vi "Dashboard Main.vi"() -> ()   [LabVIEW 2018]
uses:
  <vilib>/Utility/miscctls.llb/LVRowAndColumnTypeDef.ctl
  <vilib>/event_ctls.llb/eventvkey.ctl
  <vilib>/Rock Robotics/Network Tables/NT Read Boolean.vi
  <vilib>/Rock Robotics/Network Tables/NT Write Boolean.vi
  <vilib>/Rock Robotics/Network Tables/NT Read Numeric Array.vi
  <vilib>/Rock Robotics/WPI/Dashboard/WPI_DashboardLogging Global.vi
panel:
  in  "Camera Settings Right":T1={"Frame Rate"=30, "Compression"=30, "Size"=1, "DB Camera Config"=FALSE} {"Frame Rate" scale=1.0..30.0; "Compression" scale=100.0..-1.0; "Size" items=["640x480", "320x240", "160x120"]}
  in  "Camera Name Right":string(combo)="No Camera Selection"
  out "Camera Perf":string
  in  "Camera Settings":T1={"Frame Rate"=30, "Compression"=30, "Size"=1, "DB Camera Config"=FALSE} {"Frame Rate" scale=1.0..30.0; "Compression" scale=100.0..-1.0; "Size" items=["640x480", "320x240", "160x120"]}
  in  "TCP":refnum<k5>
  in  "Rec Mode":enum32{"Stop", "Record", "Playback"}(radio)
  out "Image Message":string="Timeout in Camera Communications"
  in  "Dashboard Tab":T2(tab)
  out "Lift Height":dbl
  in  "Auto Side":bool
  out "Limelight Target State":bool
  out "Hatch Open":bool
  out "Hatch Extend":bool
  out "Cargo Piston":bool
  in  "Zero Yaw":bool
  out "Yaw":dbl
  out "Cont Yaw":dbl
  out "LowerLimit":bool
  out "UpperLimit":bool
  out "HAB Retracting limit":bool
  out "HAB Extending limit":bool
  in  "Select Auto":string(combo)="Select Autonomous ..."
  out "NT Connection":bool
  out "Mode":T3(ring)=enum."Auto Disabled"
  out "Right Camera Perf":cluster{"Bandwidth (Mbps)":dbl, "FPS":dbl}
  out "Lift Auto Position":u16(ring) items=["Cargo 1", "Hatch 1", "Cargo 2", "Hatch 2", "Cargo 3", "Hatch 3"]
  out "CargoLimit":bool
  out "Wheel Rates":T4
  out "Wheel Angles":T4
  out "Y-Velocity":dbl
  out "X-Velocity":dbl
  out "Wheel Positions":T4
  in  "Starting Location":u16(ring)=2 items=["Left", "Center", "Right"]
  out "Positions":cluster{"X":dbl, "Y":dbl}
  out "Graph 2":cluster{cluster{"X":dbl, "Y":dbl}[]}[](graph)=[{[{"X"=44.0, "Y"=76.0}, {"X"=44.0, "Y"=76.0}]}, {[{"X"=30.03458329904793, "Y"=57.973155118857626}, {"X"=30.03458329904793, "Y"=57.973155118857626}]}, {[{"X"=29.965468303127132, "Y"=93.97308877320398}, {"X"=29.965468303127132, "Y"=93.97308877320398}]}, {[{"X"=57.96541670095207, "Y"=94.02684488114238}, {"X"=57.96541670095207, "Y"=94.02684488114238}]}, {[{"X"=58.03453169687287, "Y"=58.026911226796024}, {"X"=58.03453169687287, "Y"=58.026911226796024}]}, {[{"X"=43.942404170066, "Y"=105.9999447119553}, {"X"=43.942404170066, "Y"=105.9999447119553}]}]
  out "Tree":string(tree)
  in  "Test Slider":dbl(slide) scale=0.0..100.0 scale format="%#_3g"
  in  "On/Off":bool caption="Solenoid"
  in  "Test Name":u16(ring) items=["Select the test to run..."]
  in  "Test Tree":string(tree)
  in  "Motor":cluster{"Value":dbl, "Enable":bool} {"Value" scale=-1.0..1.0 scale format="%#_3g"}
  out "Progress":T5 {"Test Progress" scale=0.0..100.0}
  in  "Rev/Fwd":cluster{"Forward":bool, "Reverse":bool}
  in  "Test Ring":u16(ring) items=["Monochrome", "Color"]
  in  "CheckList":i32(listbox)
  out "Cmd Status":string
  in  "Execute Command":bool
  in  "Command Params":string[][](table)
  in  "Command Selection":i32(listbox)
  out "Camera Image":T6(plugin-control)
  in  "Camera Name":string(combo)="No Camera Selection"
  # "HW"
  # "HW"
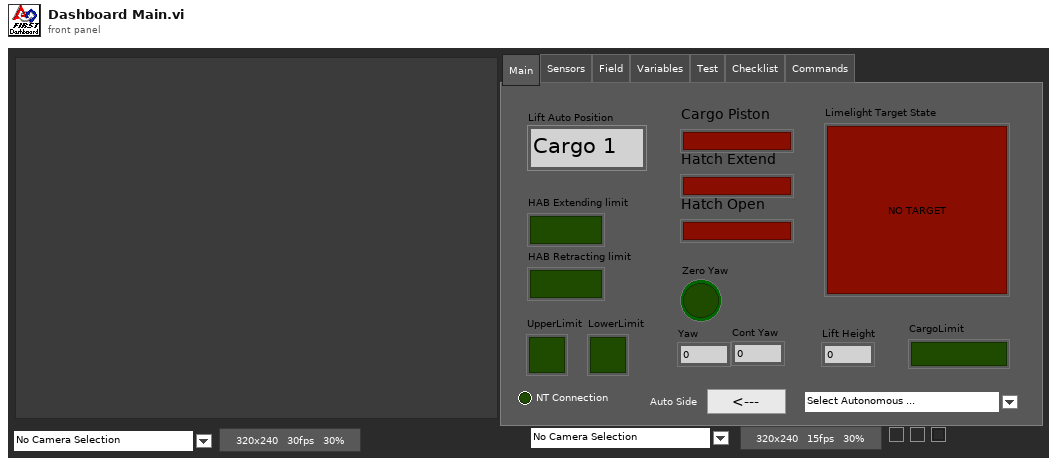
[diagram p1: front panel]
types:
  T1 = cluster{"Frame Rate":i32, "Compression":i32, "Size":u16, "DB Camera Config":bool}
  T2 = enum32{"Main", "Sensors", "Field", "Variables", "Test", "Checklist", "Commands"}
  T3 = enum8{"Tele-Op Disabled", "Tele-Op Enabled", "Auto Disabled", "Auto Enabled", "Test Disabled", "Test Enabled", "Disconnected", "No Code", "E-Stop"}
  T4 = cluster{"FrontLeft":dbl, "FrontRight":dbl, "BackLeft":dbl, "BackRight":dbl}
  T5 = cluster{"Test Progress":u8, "Test Progress Text":string}
  T6 = typedef "IMAQ Image.ctl" = refnum<image>
  T7 = cluster{"Save Path":path, "Interval (s)":dbl, "Keep":i32}
  T8 = enum32{"Drive", "Camera", "Basic", "Custom", "Test", "Commands", "Checklist", "Variables"}
  T9 = typedef "Image Type" = u32
  T10 = cluster{"IDs":cluster{"RPC field ID":u16, "Unique ID":u16}, "String":string}
  T11 = cluster{"Error Strings":string, "Disable Counts":cluster{u16, u16}, "Rail Faults":cluster{u16, u16, u16}, "Robot IP":string, "DB Mode":u8, "Event Info":cluster{"Name":string, "Type":u8, "Number":u16, "Replay":u8}}
  T12 = cluster{"Storage":cluster{"Disk Free":u64, "RAM Block":u32, "RAM free":u32}, "CPU Utilization":cluster{"CPU % ISR":sgl, "CPU % Time Crit":sgl, "CPU % Timed Str":sgl, "CPU % High":sgl, "CPU % Above":sgl, "CPU % Normal":sgl, "CPU % Low":sgl}, "CAN":cluster{"% Bus Utilization":sgl, "Bus Off Cnt":u32, "TX_FIFO Full Cnt":u32, "Receive Error Cnt":u8, "Transmit Error Cnt":u8}, "HID":cluster{"HID Outputs":u32, "Rumble Low":u16, "Rumble High":u16}[]}
  T13 = cluster{"Status bits":cluster{"Test Mode":bool, "Autonomous":bool, "Enabled":bool, "Code Start":bool, "Brownout":bool, "Reserved 2":bool, "Reserved 3":bool, "E-Stop":bool}, "Code Trace":cluster{"Disabled":bool, "TeleOp":bool, "Auto":bool, "Test":bool}, "Controller Type":enum16{"unknown", "cRIO", "roboRio"}, "Code?":enum16{"unknown", "noCode", "code"}, "Battery V":dbl}
  T14 = cluster{"Control Bits":cluster{"TestMode":bool, "Autonomous":bool, "Enabled":bool, "FMS Present":bool, bool, bool, bool, "E-Stop":bool}, "Team Station ":u8, "Countdown":sgl, "Joystick Values":cluster{"Axes":dbl[], "Buttons":bool[], "POVs":i16[]}[]}
  T15 = cluster{"Numeric":dbl, "Numeric":dbl, "Numeric":dbl, "Numeric":dbl}
  T16 = cluster{"Global Rectangle":i32[], "Contours":cluster{"Contour Type":u32, "ROI Type":u32, "Points":i32[]}[]}
  T17 = cluster{"Camera Name":string, string, "Saved DB Images Info":cluster{"Save Path":path, "Interval (s)":dbl, "Keep":i32}}
  T18 = cluster{"Camera Name Right":string, string, "Saved DB Images Info":cluster{"Save Path":path, "Interval (s)":dbl, "Keep":i32}}
  T19 = cluster{"Operation":enum16{"Update", "Clear"}, "Color Box":u32}[]
  T20 = typedef "eventvkey.ctl" = enum16{"ASCII", "Enter", "Return", "Shift", "Ctrl", "Alt", "Cmd", "Opt", "Caps", "NumLock", "Clear", "Break", "Up", "Down", "Left", "Right", "Insert", "Delete", "Home", "End", "PageUp", "PageDown", "Escape", "Help", "Pause", "ScrollLock", "F1", "F2", "F3", "F4", "F5", "F6", "F7", "F8", "F9", "F10", "F11", "F12", "F13", "F14", "F15", "F16", "F17", "F18", "F19", "F20", "F21", "F22", "F23", "F24", "Play", "VolumeUp", "VolumeDown", "Mute", "Two Byte Char"}
  T21 = cluster{"Operation":enum16{"Update", "Clear"}, "Color Box":u32}
  T22 = typedef "LVRowAndColumnTypeDef.ctl" = cluster{"Row":i32, "Column":i32}
  T23 = cluster{"Shift":bool, "Ctrl":bool, "Alt":bool, "Cmd":bool, "Opt":bool}
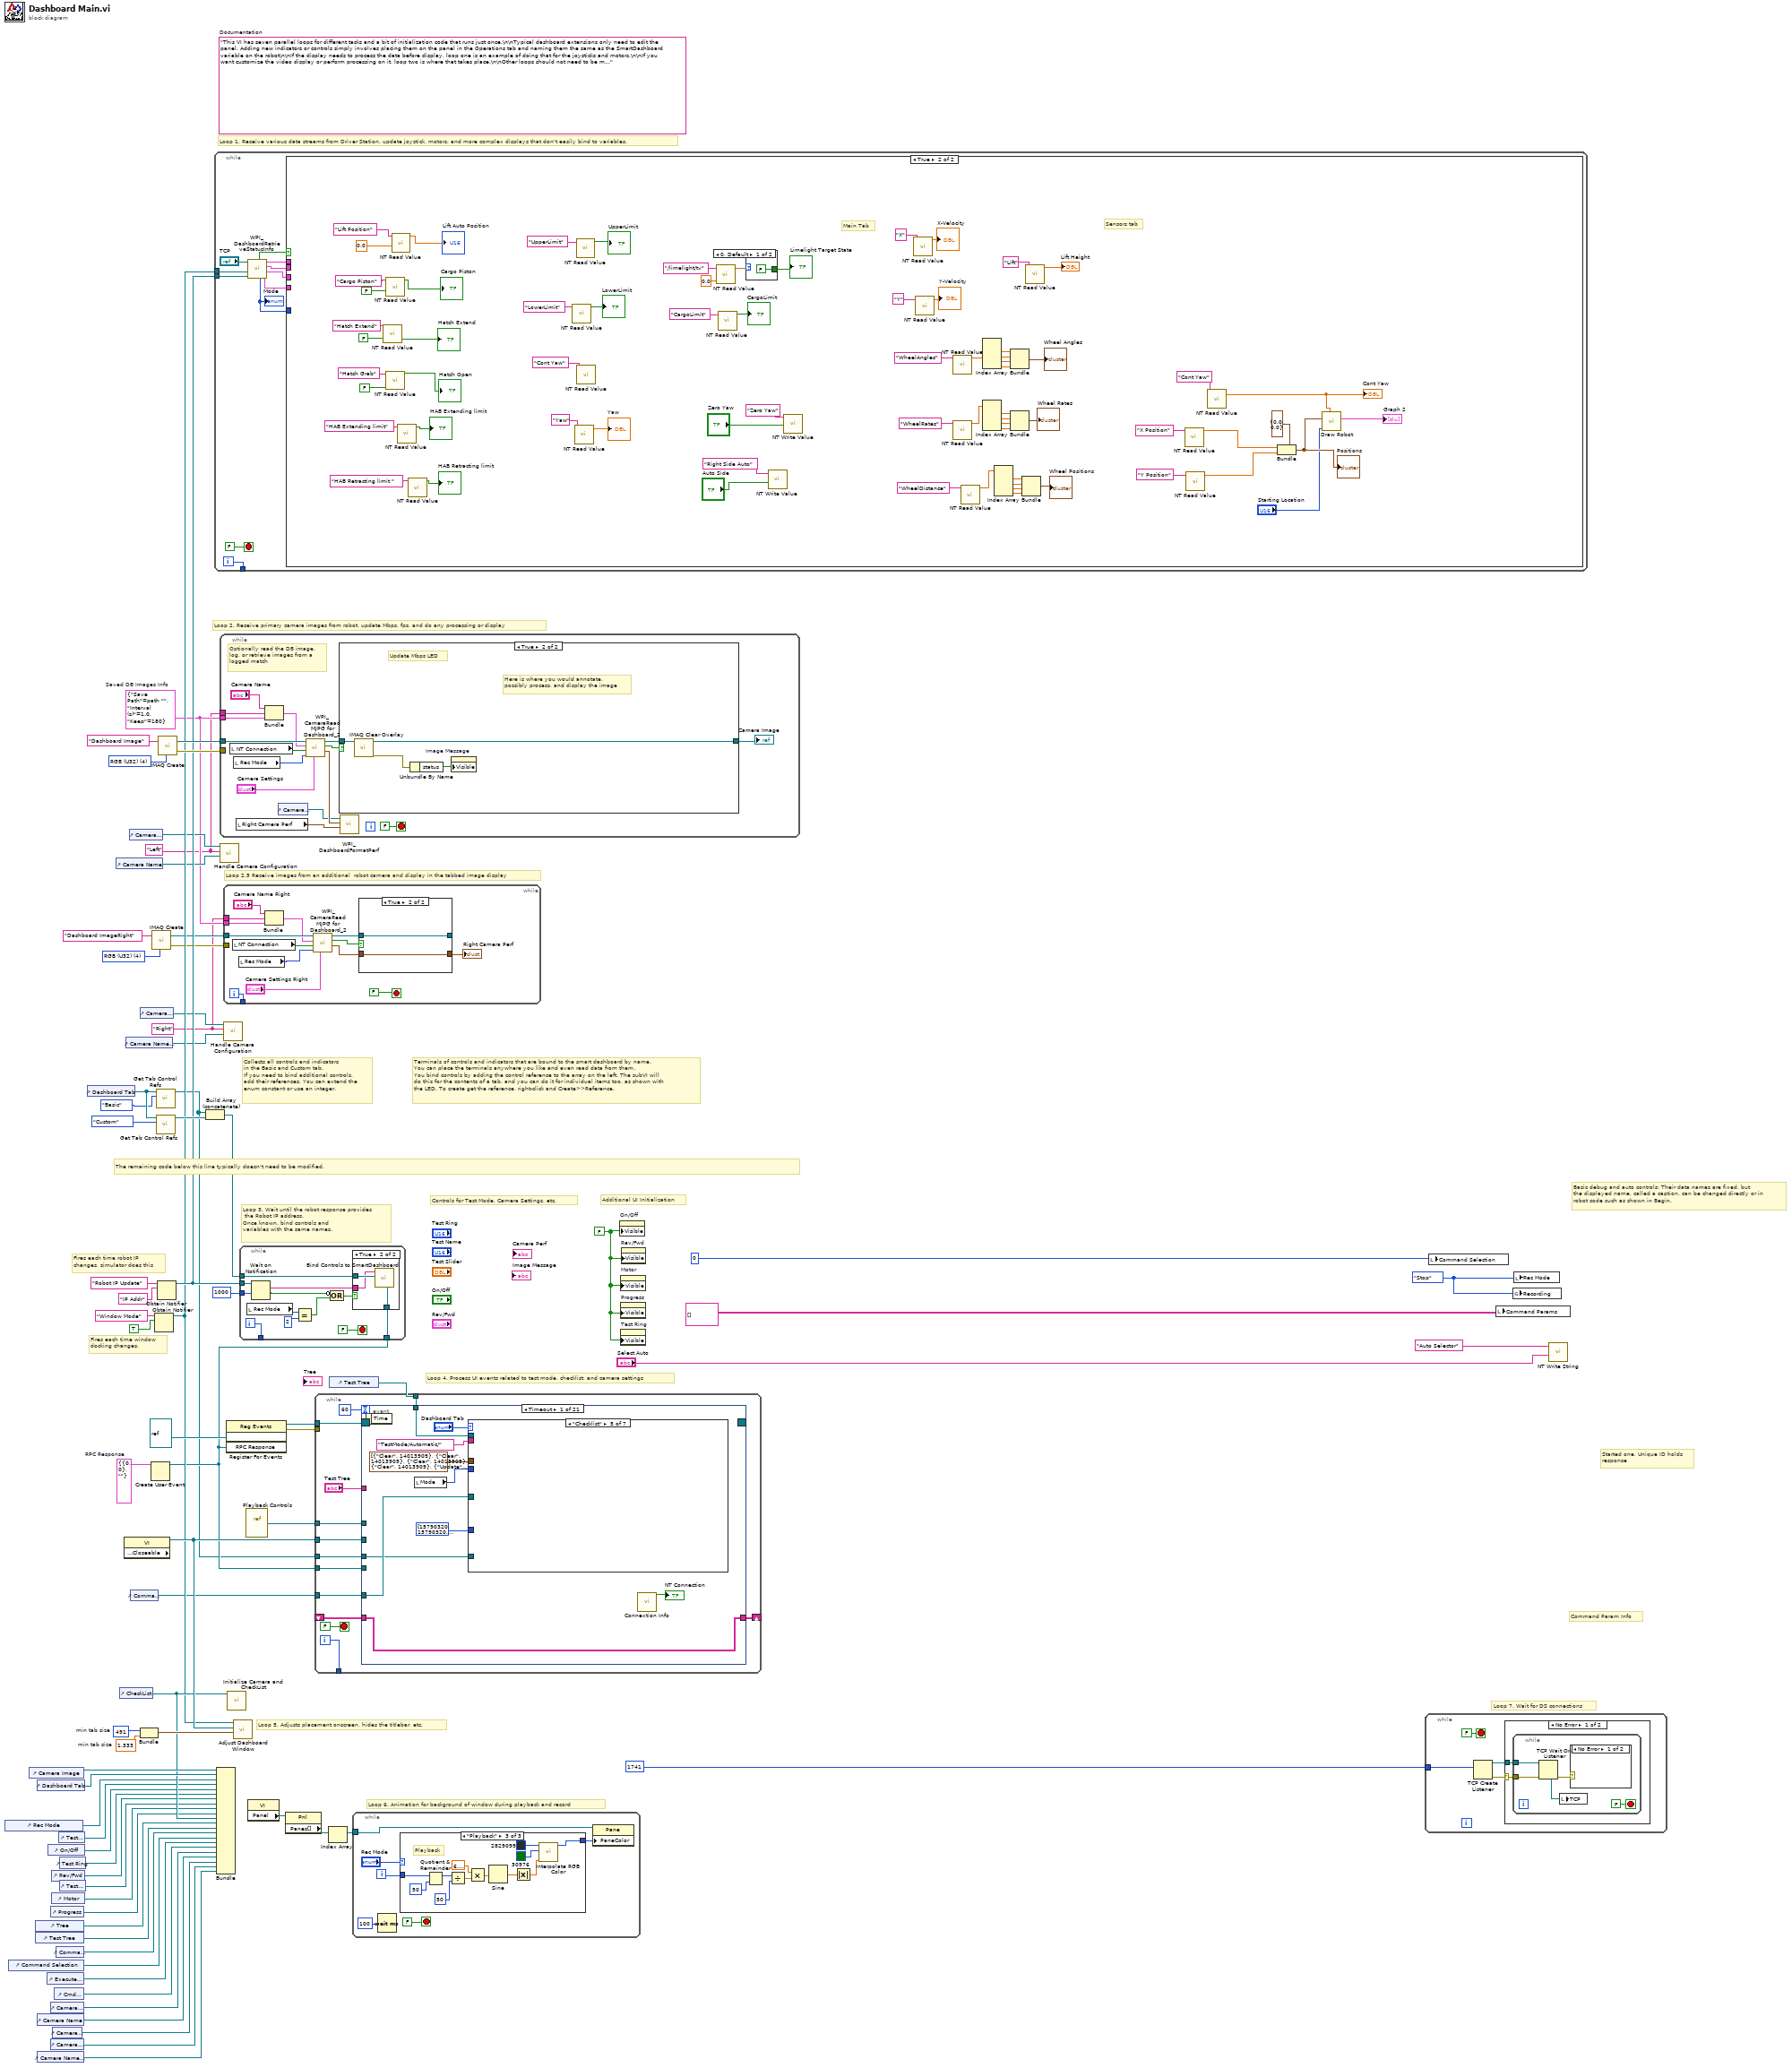
[diagram p0: block diagram]
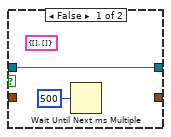
[diagram p2: hidden frame]
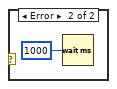
[diagram p3: hidden frame]
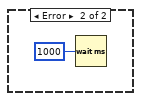
[diagram p4: hidden frame]
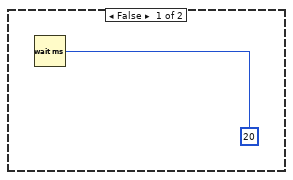
[diagram p5: hidden frame]
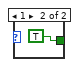
[diagram p6: hidden frame]
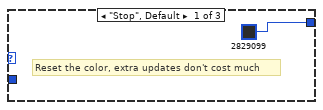
[diagram p7: hidden frame]
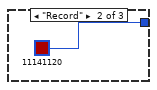
[diagram p8: hidden frame]
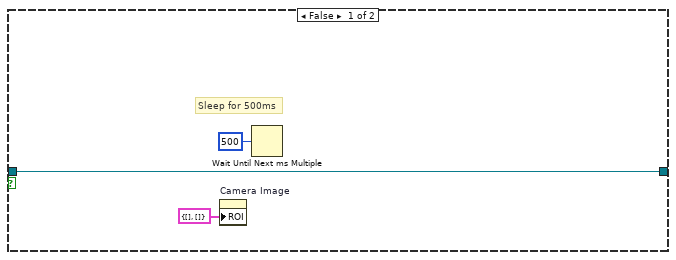
[diagram p10: hidden frame]
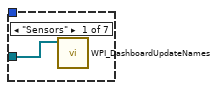
[diagram p11: hidden frame]
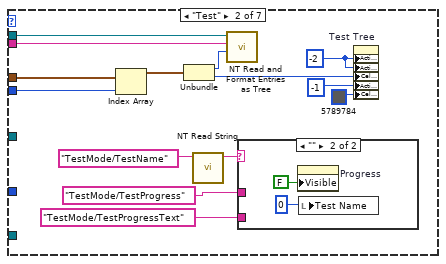
[diagram p12: hidden frame]
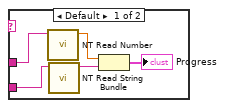
[diagram p13: hidden frame]
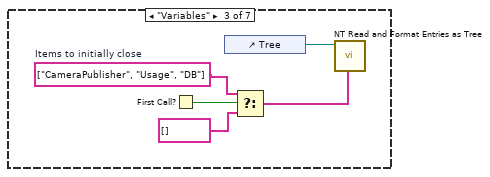
[diagram p14: hidden frame]
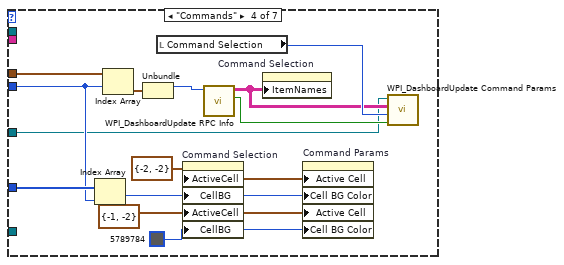
[diagram p15: hidden frame]
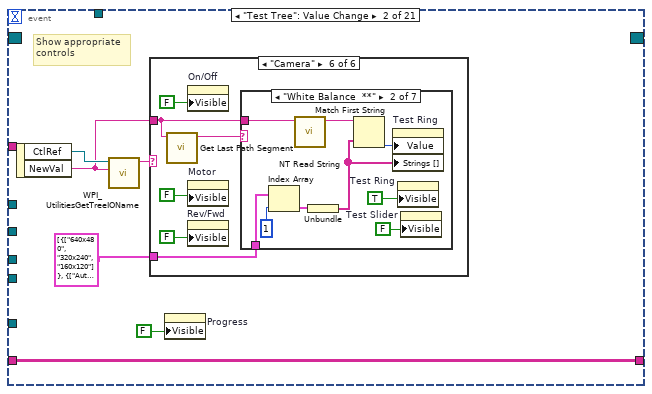
[diagram p18: hidden frame]
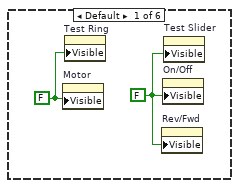
[diagram p19: hidden frame]
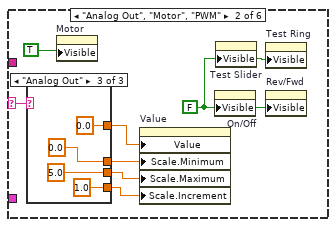
[diagram p20: hidden frame]
diagram:
  w3 = T7 {"Save Path"=path "", "Interval (s)"=1.0, "Keep"=180}  # Saved DB Images Info
  w2 = "Right"
  w1 = "Left"
  w12 = T9 4 items=["Grayscale (U8)", "Grayscale (I16)", "Grayscale (SGL)", "Complex (CSG)", "RGB (U32)", "HSL (U32)", "RGB (U64)"] ("Image Type")
  w28 = T10 {"IDs"={"RPC field ID"=0, "Unique ID"=0}, "String"=""}  # RPC Response
  w48 = 491  # min tab size
  w47 = 1.333  # min tab size
  w55 = enum32{"Stop", "Record", "Playback"}."Stop" ("Rec Mode")
  w34 = FALSE ("Visible")
  (unwired) "This VI has seven parallel loops for different tasks and a bit of initialization code that runs just once.\n\nTypical dashboard extensions only need to edit the panel. Adding new indicators or controls simply involves placing them on the panel in the Operations tab and naming them the same as the SmartDashboard variable on the robot\n\nIf the display needs to process the data before display, loop one is an example of doing that for the joysticks and motors.\n\nIf you want customize the video display or perform processing on it, loop two is where that takes place.\n\nOther loops should not need to be modified. They are pretty standard, and document the task they perform."  # Documentation
  w72 = T9 4 items=["Grayscale (U8)", "Grayscale (I16)", "Grayscale (SGL)", "Complex (CSG)", "RGB (U32)", "HSL (U32)", "RGB (U64)"] ("Image Type")
  # "Loop 2.5 Receive images from an additional  robot camera and display in the tabbed image display"
  # "Command Param Info"
  # "Started one, Unique ID holds\nresponse"
  # "Loop 7. Wait for DS connections"
  # "Basic debug and auto controls: Their data names are fixed, but\nthe displayed name, called a caption, can be changed directly or in\nrobot code such as shown in Begin."
  # "Controls for Test Mode, Camera Settings, etc."
  # "Additional UI Initialization"
  # "Loop 6. Animation for background of window during playback and record"
  # "Fires each time robot IP\nchanges, simulator does this"
  # "Fires each time window\ndocking changes."
  # "Collects all controls and indicators\nin the Basic and Custom tab.\nIf you need to bind additional controls,\nadd their references. You can extend the\nenum constant or use an integer."
  # "The remaining code below this line typically doesn't need to be modified."
  # "Loop 4. Process UI events related to test mode, checklist, and camera settings"
  # "Terminals of controls and indicators that are bound to the smart dashboard by name.\nYou can place the terminals anywhere you like and even read data from them.\nYou bind controls by adding the control reference to the array on the left. The subVI will\ndo this for the contents of a tab, and you can do it for individual items too, as shown with\nthe LED. To create get the reference, right-click and Create>>Reference."
  # "Loop 3. Wait until the robot response provides\n the Robot IP address.\nOnce known, bind controls and\nvariables with the same names."
  # "Loop 5. Adjusts placement onscreen, hides the titlebar, etc."
  # "Loop 1. Receive various data streams from Driver Station, update joystick, motors, and more complex displays that don't easily bind to variables."
  # "Loop 2. Receive primary camera images from robot, update Mbps, fps, and do any processing or display"
  n1 = control-ref of="Rec Mode"() -> (w40:refnum<vi>)
  n2 = control-ref of="Command Selection"() -> (w27:refnum<vi>)
  n3 = control-ref of="Camera Image"() -> (w50:refnum<vi>)
  n4 = control-ref of="Tree"() -> (w44:refnum<vi>)
  n5 = control-ref of="Test Tree"() -> (w43:refnum<vi>)
  n6 = control-ref of="Dashboard Tab"() -> (w49:refnum<vi>)
  n7 = control-ref of="Camera Name"() -> (w18:refnum<vi>)
  n8 = control-ref of="Camera Name Right"() -> (w6:refnum<vi>)
  n9 = control-ref of="Execute Command"() -> (w29:refnum<vi>)
  n10 = control-ref of="On/Off"() -> (w38:refnum<vi>)
  n11 = control-ref of="Progress"() -> (w35:refnum<vi>)
  n12 = control-ref of="Camera Settings"() -> (w19:refnum<vi>)
  n13 = control-ref of="Camera Settings Right"() -> (w7:refnum<vi>)
  n14 = control-ref of="Rev/Fwd"() -> (w36:refnum<vi>)
  n15 = control-ref of="Motor"() -> (w41:refnum<vi>)
  n16 = control-ref of="Camera Perf"() -> (w17:refnum<vi>)
  n17 = control-ref of="Cmd Status"() -> (w23:refnum<vi>)
  n18 = control-ref of="Command Params"() -> (w30:refnum<vi>)
  n19 = control-ref of="Test Slider"() -> (w39:refnum<vi>)
  n20 = control-ref of="Test Ring"() -> (w37:refnum<vi>)
  n21 = control-ref of="Test Name"() -> (w42:refnum<vi>)
  n22 = control-ref of="Dashboard Tab"() -> (w53:refnum<vi>)
  n23 = control-ref of="Camera Name"() -> (w20:refnum<vi>)
  n24 = control-ref of="CheckList"() -> (w45:refnum<vi>)
  n25 = property class="VI" props=["Front Panel.Closeable"]() -> (reference out=w54:refnum<vi>)  [unwired: 2 in, 2 out]
  n26 = control-ref of="Camera Name Right"() -> (w8:refnum<vi>)
  n27 = control-ref of="Camera Settings"() -> (w21:refnum<vi>)
  n28 = control-ref of="Command Params"() -> (w22:refnum<vi>)
  n29 = control-ref of="Camera Settings Right"() -> (w9:refnum<vi>)
  n30 = Bundle("min tab size"=w48, "min tab size"=w47) -> (w46:cluster{"min tab size":i32, "min tab size":dbl})  [unwired: 1 in]
  n31 = Create User Event(user event datatype=w28) -> (user event=w24:refnum<user-event>)  [unwired: 1 in, 1 out]
  n32 = call "IMAQ Create"("Image Name"="Dashboard ImageRight", "Image Type"=w12) -> ("New Image"=w11:T6, "error out"=w10:errorcluster)  [unwired: 2 in, 1 out]
  n33 = Obtain Notifier(name (unnamed)="Window Mode", notification data type=TRUE) -> (notifier out=w32:refnum<notifier>)  [unwired: 2 in, 2 out]
  n34 = call <vilib>:"Get Tab Control Refs.vi"("Page Index"=T8."Basic" ("Dashboard Tab"), "TabControl in"=w53) -> ("ControlsOnPage"=w16:refnum<vi>[])  [unwired: 9 in]
  n35 = call <vilib>:"Get Tab Control Refs.vi"("Page Index"=T8."Custom" ("Dashboard Tab"), "TabControl in"=w53) -> ("ControlsOnPage"=w52:refnum<vi>[])  [unwired: 9 in]
  n36 = Obtain Notifier(name (unnamed)="Robot IP Update", notification data type="IP Addr" ("name (unnamed)")) -> (notifier out=w33:refnum<notifier>)  [unwired: 2 in, 2 out]
  n37 = call "IMAQ Create"("Image Name"="Dashboard Image", "Image Type"=w72) -> ("New Image"=w70:T6, "error out"=w69:errorcluster)  [unwired: 2 in, 1 out]
  n38 = Build Array (concatenate)(w16, w52) -> (w51:refnum<vi>[])
  n39 = while {
    tunnel: [w82] -> _
    tunnel: w33 -> [w80]
    tunnel: w32 -> [w77]
    i -> [w82]
    stop <- FALSE stop-if-true
    n40 = call <vilib>:"WPI_DashboardRetrieveStatusInfo.vi"("Binding Refnum"=w80, "Window Mode Notifier"=w77, "TCP Cnx"="TCP") -> ("Power and Errors"=w74:T11, "Robot Metrics"=w73:T12, "Status Info"=w75:T13, "Control Info"=w76:T14, "Robot Mode"=w79:T3, "Process?"=w81:bool)  [unwired: 3 in]
    "Mode" <- w79
    n41 = case shown="True" w81 {
      tunnel: w79 -> [_ _]
      tunnel: w76 -> [_ _]
      tunnel: w75 -> [_ _]
      tunnel: w74 -> [_ _]
      tunnel: w73 -> [_ _]
      frame False {
        n42 = Wait (ms)(milliseconds to wait=u32 20) -> ()  [unwired: 1 out]
      }
      frame True {
        # "Sensors tab"
        # "Main Tab"
        n43 = call-poly <vilib>:"NT Read Value.vi"("Default Value"=FALSE, "Name"="Hatch Extend") -> ("Boolean"=→"Hatch Extend":bool)  [unwired: 8 in, 1 out]
        n44 = call-poly <vilib>:"NT Read Value.vi"("Default Value"=FALSE, "Name"="Cargo Piston") -> ("Boolean"=→"Cargo Piston":bool)  [unwired: 8 in, 1 out]
        n45 = call-poly <vilib>:"NT Read Value.vi"("Default Value"=FALSE, "Name"="Hatch Grab") -> ("Boolean"=→"Hatch Open":bool)  [unwired: 8 in, 1 out]
        n46 = call-poly <vilib>:"NT Read Value.vi"("Default Value"=0.0, "Name"="Lift Position") -> ("Numeric"=→"Lift Auto Position":dbl)  [unwired: 8 in, 1 out]
        n47 = call-poly <vilib>:"NT Read Value.vi"("Name"="HAB Extending limit") -> ("Boolean"=→"HAB Extending limit":bool)  [unwired: 9 in, 1 out]
        n48 = call-poly <vilib>:"NT Read Value.vi"("Name"="HAB Retracting limit ") -> ("Boolean"=→"HAB Retracting limit":bool)  [unwired: 9 in, 1 out]
        n49 = call-poly <vilib>:"NT Read Value.vi"("Name"="LowerLimit") -> ("Boolean"=→"LowerLimit":bool)  [unwired: 9 in, 1 out]
        n50 = call-poly <vilib>:"NT Read Value.vi"("Name"="Yaw") -> ("Numeric"=→"Yaw":dbl)  [unwired: 9 in, 1 out]
        n51 = call-poly <vilib>:"NT Read Value.vi"("Name"="UpperLimit") -> ("Boolean"=→"UpperLimit":bool)  [unwired: 9 in, 1 out]
        n52 = call-poly <vilib>:"NT Read Value.vi"("Name"="Cont Yaw") -> ()  [unwired: 9 in, 2 out]
        n53 = call-poly <vilib>:"NT Read Value.vi"("Default Value"=0.0, "Name"="/limelight/tv") -> ("Numeric"=w122:dbl)  [unwired: 8 in, 1 out]
        n54 = call-poly <vilib>:"NT Read Value.vi"("Name"="CargoLimit") -> ("Boolean"=→"CargoLimit":bool)  [unwired: 9 in, 1 out]
        n55 = case shown="0, Default" w122 {
          tunnel: [FALSE TRUE] -> w121
          frame 0, Default {
          }
          frame 1 {
          }
        }
        "Limelight Target State" <- w121
        n56 = call-poly <vilib>:"NT Write Value.vi"("Boolean"="Auto Side", "Name"="Right Side Auto") -> ()  [unwired: 9 in, 1 out]
        n57 = call-poly <vilib>:"NT Write Value.vi"("Boolean"="Zero Yaw", "Name"="Zero Yaw") -> ()  [unwired: 9 in, 1 out]
        n58 = call-poly <vilib>:"NT Read Value.vi"("Name"="X") -> ("Numeric"=→"X-Velocity":dbl)  [unwired: 9 in, 1 out]
        n59 = call-poly <vilib>:"NT Read Value.vi"("Name"="Y") -> ("Numeric"=→"Y-Velocity":dbl)  [unwired: 9 in, 1 out]
        n60 = call-poly <vilib>:"NT Read Value.vi"("Name"="WheelAngles") -> ("Numeric Array"=w119:dbl[])  [unwired: 9 in, 1 out]
        n61 = call-poly <vilib>:"NT Read Value.vi"("Name"="WheelRates") -> ("Numeric Array"=w109:dbl[])  [unwired: 9 in, 1 out]
        n62 = call-poly <vilib>:"NT Read Value.vi"("Name"="WheelDistance") -> ("Numeric Array"=w104:dbl[])  [unwired: 9 in, 1 out]
        n63 = Index Array(array=w119) -> (element #1=w118:dbl, element #2=w117:dbl, element #3=w116:dbl, element #4=w115:dbl)  [unwired: 4 in]
        n64 = Index Array(array=w109) -> (element #1=w110:dbl, element #2=w111:dbl, element #3=w112:dbl, element #4=w113:dbl)  [unwired: 4 in]
        n65 = Index Array(array=w104) -> (element #1=w103:dbl, element #2=w102:dbl, element #3=w101:dbl, element #4=w100:dbl)  [unwired: 4 in]
        n66 = Bundle("Numeric"=w118, "Numeric"=w117, "Numeric"=w116, "Numeric"=w115) -> (→"Wheel Angles":T15)  [unwired: 1 in]
        n67 = Bundle("Numeric"=w110, "Numeric"=w111, "Numeric"=w112, "Numeric"=w113) -> (→"Wheel Rates":T15)  [unwired: 1 in]
        n68 = Bundle("Numeric"=w103, "Numeric"=w102, "Numeric"=w101, "Numeric"=w100) -> (→"Wheel Positions":T15)  [unwired: 1 in]
        n69 = call-poly <vilib>:"NT Read Value.vi"("Name"="Lift") -> ("Numeric"=→"Lift Height":dbl)  [unwired: 9 in, 1 out]
        n70 = call-poly <vilib>:"NT Read Value.vi"("Name"="X Position") -> ("Numeric"=w86:dbl)  [unwired: 9 in, 1 out]
        n71 = call-poly <vilib>:"NT Read Value.vi"("Name"="Y Position") -> ("Numeric"=w87:dbl)  [unwired: 9 in, 1 out]
        n72 = call-poly <vilib>:"NT Read Value.vi"("Name"="Cont Yaw") -> ("Numeric"=w90:dbl)  [unwired: 9 in, 1 out]
        "Cont Yaw" <- w90
        n73 = Bundle(cluster=cluster{"Numeric":dbl, "Numeric":dbl} {"Numeric"=0.0, "Numeric"=0.0}, "Numeric"=w86, "Numeric"=w87) -> (w93:cluster{"Numeric":dbl, "Numeric":dbl})
        "Positions" <- w93
        n74 = call "Draw Robot.vi"("Gyro"=w90, "Starting Location"="Starting Location", "XY"=w93) -> ("Graph 2"=→"Graph 2":cluster{cluster{"X":dbl, "Y":dbl}[]}[])  [unwired: 8 in]
      }
    }
  }
  n75 = Bundle("Camera Image"=w50, "Dashboard Tab"=w49, "Rec Mode"=w40, "Test Slider"=w39, "On/Off"=w38, "Test Ring"=w37, "Rev/Fwd"=w36, "Test Name"=w42, "Motor"=w41, "Progress"=w35, "CheckList"=w45, "Tree"=w44, "Test Tree"=w43, "Command Params"=w30, "Command Selection"=w27, "Execute Command"=w29, "Cmd Status"=w23, "Camera Settings"=w19, "Camera Name"=w18, "Camera Perf"=w17, "Camera Settings Right"=w7, "Camera Name Right"=w6) -> ()  [unwired: 1 in, 1 out]
  n76 = call "Handle Camera Configuration.vi"("CameraNameRef"=w20, "Display Name"=w1, "ClusterRef"=w21) -> ()  [unwired: 9 in]
  n77 = while {
    tunnel: w70 -> [w170]
    tunnel: w69 -> [_]
    tunnel: w3 -> [w163]
    tunnel: w1 -> [w160]
    stop <- FALSE stop-if-true
    # "Optionally read the DB image,\nlog, or retrieve images from a\nlogged match"
    n78 = local read "NT Connection"() -> (w164:bool)
    n79 = local read "Rec Mode"() -> (w167:enum32{"Stop", "Record", "Playback"})
    n80 = local read "Right Camera Perf"() -> (w158:cluster{"Bandwidth (Mbps)":dbl, "FPS":dbl})
    n81 = Bundle("Camera Name"="Camera Name", w160, "Saved DB Images Info"=w163) -> (w162:T17)  [unwired: 1 in]
    n82 = control-ref of="Camera Perf"() -> (w157:refnum<vi>)
    n83 = call <vilib>:"WPI_CameraRead MJPG for Dashboard_2.vi"("Camera Settings"="Camera Settings", "Rec Mode"=w167, "NT Connection"=w164, "Capture Info"=w162, "Image in"=w170) -> ("perf info"=w159:cluster{"Bandwidth (Mbps)":dbl, "fps":dbl}, "Active"=w168:bool, "Image\\ out"=w169:T6)  [unwired: 4 in]
    n84 = case shown="True" w168 {
      tunnel: w169 -> [w173 w176]
      tunnel: [w173 w175] -> w165
      frame False {
        # "Sleep for 500ms"
        n85 = property on="Camera Image" class="ImageControl"("ROI"=T16 {"Global Rectangle"=[], "Contours"=[]}) -> ()  [unwired: 2 in, 2 out]
        n86 = Wait Until Next ms Multiple(millisecond multiple=u32 500) -> ()  [unwired: 1 out]
      }
      frame True {
        # "Here is where you would annotate,\npossibly process, and display the image"
        # "Update Mbps LED"
        n87 = call "IMAQ Clear Overlay"("Image"=w176) -> ("error out"=w177:errorcluster, "Image Out"=w175:T6)  [unwired: 2 in, 7 out]
        n88 = Unbundle By Name(w177) -> ("status"=w178:bool)
        n89 = property on="Image Message" class="Str"("Visible"=w178) -> ()  [unwired: 2 in, 2 out]
      }
    }
    "Camera Image" <- w165
    n90 = call <vilib>:"WPI_DashboardFormatPerf.vi"("Right Camera Perf"=w158, "Performance"=w159, "String in"=w157) -> ()  [unwired: 9 in]
  }
  n91 = call "Handle Camera Configuration.vi"("CameraNameRef"=w8, "Display Name"=w2, "ClusterRef"=w9) -> ()  [unwired: 9 in]
  n92 = while {
    tunnel: w11 -> [w192]
    tunnel: w10 -> [_]
    tunnel: [w187] -> _
    tunnel: w3 -> [w184]
    tunnel: w2 -> [w181]
    i -> [w187]
    stop <- FALSE stop-if-true
    n93 = local read "NT Connection"() -> (w185:bool)
    n94 = local read "Rec Mode"() -> (w191:enum32{"Stop", "Record", "Playback"})
    n95 = Bundle("Camera Name Right"="Camera Name Right", w181, "Saved DB Images Info"=w184) -> (w183:T18)  [unwired: 1 in]
    n96 = call <vilib>:"WPI_CameraRead MJPG for Dashboard_2.vi"("Camera Settings"="Camera Settings Right", "Rec Mode"=w191, "NT Connection"=w185, "Capture Info"=w183, "Image in"=w192) -> ("perf info"=w179:cluster{"Bandwidth (Mbps)":dbl, "fps":dbl}, "Active"=w186:bool, "Image\\ out"=w189:T6)  [unwired: 4 in]
    n97 = case shown="True" w186 {
      tunnel: w189 -> [w193 w196]
      tunnel: [w193 w196] -> _
      tunnel: [_ w195] -> w180
      tunnel: w179 -> [_ w195]
      frame False {
        (unwired) T16 {"Global Rectangle"=[], "Contours"=[]} ("ROI")
        n98 = Wait Until Next ms Multiple(millisecond multiple=u32 500) -> ()  [unwired: 1 out]
      }
      frame True {
      }
    }
    "Right Camera Perf" <- w180
  }
  n99 = register-events(refnum<vi> refnum, w24) -> (reference out=w59:refnum<event-registration>, error out=w58:errorcluster)  [unwired: 2 in]
  n100 = call "Initialize Camera and CheckList.vi"("ListBox in"=w45) -> ()  [unwired: 11 in]
  n101 = call "Adjust Dashboard Window.vi"("Size Constraints"=w46, "VI"=w54, "WIn Mode"=w32) -> ()  [unwired: 9 in]
  n102 = while {
    tunnel: w51 -> [w208]
    tunnel: w33 -> [w206]
    tunnel: [w204] -> _
    tunnel: u32 1000 ("milliseconds to wait") -> [w203]
    tunnel: w24 -> [w197]
    i -> [w204]
    stop <- FALSE stop-if-true
    n103 = local read "Rec Mode"() -> (w199:enum32{"Stop", "Record", "Playback"})
    n104 = Wait on Notification(notifier=w206, timeout in ms (-1)=w203) -> (notification=w205:string, timed out?=w201:bool)  [unwired: 2 in, 2 out]
    n105 = Equal?(x=w199, y=u16 2 ("Rec Mode")) -> (x = y?=w200:bool)
    n106 = Compound Arithmetic op=OR(invert w201, w200) -> (w202:bool)
    n107 = case shown="True" w202 {
      tunnel: w208 -> [_ w211]
      tunnel: w205 -> [_ w210]
      tunnel: w197 -> [_ w209]
      frame False {
      }
      frame True {
        n108 = call <vilib>:"Bind Controls to SmartDashboard.vi"("RPC ref"=w209, "Bound Control Refs"=w211, "Server IP Address"=w210) -> ()  [unwired: 9 in]
      }
    }
  }
  n109 = vi-ref "Playback Controls.vi"() -> (w60:refnum<vi>)
  n110 = property class="VI"() -> ("Panel"=w62:refnum<vi>)  [unwired: 2 in, 2 out]
  n111 = property class="Pnl"(reference=w62) -> ("Panes[]"=w63:refnum<vi>[])  [unwired: 1 in, 2 out]
  n112 = Index Array(array=w63) -> (element=w61:refnum<vi>)  [unwired: 1 in]
  n113 = control-ref of="Test Tree"() -> (w64:refnum<vi>)
  n114 = while {
    tunnel: [w221] -> _
    tunnel: w64 -> [w220]
    tunnel: w60 -> [w219]
    tunnel: w59 -> [w218]
    tunnel: w58 -> [_]
    tunnel: w54 -> [w217]
    tunnel: w24 -> [w216]
    tunnel: w22 -> [w215]
    shift-right: [w214] -> _
    shift-left: _ -> [w213]
    tunnel: w16 -> [w212]
    i -> [w221]
    stop <- FALSE stop-if-true
    n115 = event shown="[0] Timeout" {
      selector: w218 -> [_ _ _ _ _ _ _ _ _ _ _ _ _ _ _ _ _ _ _ _ _]
      dyn-events: [_ _ _ _ _ _ _ _ _ _ _ _ _ _ _ _ w479 _ _ _ _] -> _
      timeout: u32 60 ("milliseconds to wait") -> [_ _ _ _ _ _ _ _ _ _ _ _ _ _ _ _ _ _ _ _ _]
      tunnel: w220 -> [w233 _ _ _ _ _ _ _ _ _ _ _ _ _ _ _ _ _ _ _ _]
      tunnel: "Test Tree" -> [_ _ _ _ _ _ _ _ _ _ _ w448 w456 w458 w462 w470 _ _ _ _ _]
      tunnel: w219 -> [_ _ _ _ _ _ _ _ _ _ _ _ _ _ _ _ w481 _ w497 _ _]
      tunnel: w217 -> [_ _ _ _ _ _ _ _ _ _ _ _ _ _ _ _ w477 _ _ _ _]
      tunnel: w216 -> [_ _ _ _ _ _ _ _ _ _ _ _ _ _ _ _ w475 _ _ _ _]
      tunnel: w215 -> [w228 _ _ _ _ _ w399 _ _ _ _ _ _ _ _ _ _ _ _ _ _]
      tunnel: [w227 w276 w378 w383 w392 w396 w397 w406 w416 w423 w435 w447 w454 w457 w461 w469 w474 w492 w494 w498 w511] -> w214
      tunnel: w213 -> [w227 w276 w378 w383 w392 w396 w397 _ _ w423 w435 w447 w454 w457 w461 w469 w474 w492 w494 w498 w511]
      tunnel: w212 -> [w225 _ _ _ _ _ _ _ _ _ _ _ _ _ _ _ _ _ _ _ _]
      event Timeout {
        n116 = event-data() -> ()  [unwired: 1 in, 1 out]
        n117 = local read "Mode"() -> (w230:T3)
        n118 = case shown="\"Checklist\"" "Dashboard Tab" {
          tunnel: w233 -> [_ w249 _ _ _ _ _]
          tunnel: "TestMode/Automatic/" ("Name Pattern") -> [_ w248 _ _ _ _ _]
          tunnel: T19 [{"Operation"=enum."Clear", "Color Box"=14013909}, {"Operation"=enum."Clear", "Color Box"=14013909}, {"Operation"=enum."Clear", "Color Box"=14013909}, {"Operation"=enum."Clear", "Color Box"=14013909}, {"Operation"=enum."Update", "Color Box"=14013909}, {"Operation"=enum."Update", "Color Box"=16777215}, {"Operation"=enum."Clear", "Color Box"=14013909}, {"Operation"=enum."Clear", "Color Box"=14013909}, {"Operation"=enum."Clear", "Color Box"=14013909}] -> [_ w241 _ w269 _ _ _]
          tunnel: w230 -> [_ w240 _ w268 _ _ _]
          tunnel: u32[] [15790320, 15790320, 15790320, 15790320, 16777215, 16777215, 15790320, 15790320, 15790320] -> [_ _ _ w274 _ _ _]
          tunnel: w228 -> [_ _ _ w262 _ _ _]
          tunnel: w225 -> [w235 _ _ _ _ _ _]
          frame "Sensors" {
            n119 = call <vilib>:"WPI_DashboardUpdateNames.vi"("Controls on Tab"=w235) -> ()  [unwired: 11 in]
          }
          frame "Test" {
            w247 = -2 ("Active Item:Row Number")
            n120 = Index Array(array=w241, index=w240) -> (element=w242:T21)
            n121 = Unbundle(w242) -> ("Operation"=w243:enum16{"Update", "Clear"}, "Color Box"=w244:u32)
            n122 = call <vilib>:"NT Read String.vi"("Name"="TestMode/TestName") -> ("String"=w238:string)  [unwired: 9 in, 1 out]
            n123 = call <vilib>:"NT Read and Format Entries as Tree.vi"("Operation"=w243, "Name Pattern"=w248, "Tree Refnum"=w249) -> ()  [unwired: 7 in, 2 out]
            n124 = case shown="\"\"" w238 {
              tunnel: "TestMode/TestProgress" ("Name") -> [w251 _]
              tunnel: "TestMode/TestProgressText" ("Name") -> [w250 _]
              frame Default {
                n125 = call <vilib>:"NT Read Number.vi"("Name"=w251) -> ("Numeric"=w252:dbl)  [unwired: 9 in, 1 out]
                n126 = call <vilib>:"NT Read String.vi"("Name"=w250) -> ("String"=w253:string)  [unwired: 9 in, 1 out]
                n127 = Bundle("Numeric"=w252, "String"=w253) -> (→"Progress":cluster{"Numeric":dbl, "String":string})  [unwired: 1 in]
              }
              frame "" {
                n128 = property on="Progress" class="Clust (strict)"("Visible"=FALSE) -> ()  [unwired: 2 in, 2 out]
                n129 = local write "Test Name"(u16 0) -> ()
              }
            }
            n130 = property on="Test Tree" class="Tree (strict)"("Active Item Row Number"=w247, "ActiveColNum"=w247, "CellBG"=w244, "Active Item Row Number"=-1 ("Active Item:Row Number"), "CellBG"=u32 5789784 ("Color Box")) -> ()  [unwired: 2 in, 2 out]
          }
          frame "Variables" {
            w259 = string[] ["CameraPublisher", "Usage", "DB"]  # Items to initially close
            n131 = First Call?() -> (First Call?: T/F=w260:bool)
            n132 = control-ref of="Tree"() -> (w261:refnum<vi>)
            n133 = Select(t=w259, s=w260, f=string[] []) -> (s? t:f=w257:string[])
            n134 = call <vilib>:"NT Read and Format Entries as Tree.vi"("Tags to  Close"=w257, "Tree Refnum"=w261) -> ()  [unwired: 8 in, 2 out]
          }
          frame "Commands" {
            w270 = u32 5789784 ("Color Box")
            w271 = T22 {"Row"=-1, "Column"=-2} ("Active Cell:Active Cell")
            w273 = T22 {"Row"=-2, "Column"=-2} ("Active Cell:Active Cell")
            n135 = Index Array(array=w274, index=w268) -> (element=w272:u32)
            n136 = Index Array(array=w269, index=w268) -> (element=w267:T21)
            n137 = Unbundle(w267) -> ("Operation"=w266:enum16{"Update", "Clear"})  [unwired: 1 out]
            n138 = local read "Command Selection"() -> (w265:i32)
            n139 = property on="Command Selection" class="MCListbox (strict)"("ActiveCell"=w273, "CellBG"=w272, "ActiveCell"=w271, "CellBG"=w270) -> ()  [unwired: 2 in, 2 out]
            n140 = call <vilib>:"WPI_DashboardUpdate RPC Info.vi"("Operation"=w266) -> ("update"=w264:bool, "commands"=w263:string[][])  [unwired: 9 in]
            n141 = property on="Command Selection" class="MCListbox (strict)"("ItemNames"=w263) -> ()  [unwired: 2 in, 2 out]
            n142 = property on="Command Params" class="Tbl (strict)"("Active Cell"=w273, "Cell BG Color"=w272, "Active Cell"=w271, "Cell BG Color"=w270) -> ()  [unwired: 2 in, 2 out]
            n143 = call <vilib>:"WPI_DashboardUpdate Command Params.vi"("Update"=w264, "NewVal"=w265, "Commands"=w263, "Param Tbl"=w262) -> ()  [unwired: 7 in, 1 out]
          }
          frame "Checklist" {
          }
          frame "Main" {
          }
          frame "Field" {
          }
        }
        n144 = call <vilib>:"Connextion Info.vi"() -> ("Connected"=→"NT Connection":bool)  [unwired: 10 in, 1 out]
      }
      event "Test Tree": Value Change {
        # "Show appropriate\ncontrols"
        n145 = event-data() -> ("CtlRef"=w279:refnum<vi>, "NewVal"=w277:string)  [unwired: 1 in]
        n146 = call <vilib>:"WPI_UtilitiesGetTreeIOName.vi"("NewVal"=w277, "TreeControl in"=w279) -> ("I/O Name"=w280:string)  [unwired: 9 in]
        n147 = case shown="\"Camera\"" w280 {
          selector: w280 -> [_ w287 _ w309 w318 _]
          tunnel: w277 -> [_ _ w306 w308 _ w325]
          tunnel: cluster{string[]}[] [{["640x480", "320x240", "160x120"]}, {["Auto", "Fixed indoor", "Fixed outdoor 1", "Fixed outdoor 2", "Fixed fluorescent 1", "Fixed fluorescent 2", "Hold current"]}, {["Auto", "Flicker-free 50 Hz", "Flicker-free 60 Hz", "Hold current"]}, {["None", "Prioritize frame rate", "Prioritize image quality"]}, {["Monochrome", "Color"]}] -> [_ _ _ _ _ w324]
          frame Default {
            w282 = FALSE ("Visible")
            w281 = FALSE ("Visible")
            n148 = property on="Motor" class="Clust (strict)"("Visible"=w281) -> ()  [unwired: 2 in, 2 out]
            n149 = property on="Test Ring" class="Ring (strict)"("Visible"=w281) -> ()  [unwired: 2 in, 2 out]
            n150 = property on="Rev/Fwd" class="Clust (strict)"("Visible"=w282) -> ()  [unwired: 2 in, 2 out]
            n151 = property on="On/Off" class="Bool (strict)"("Visible"=w282) -> ()  [unwired: 2 in, 2 out]
            n152 = property on="Test Slider" class="Slide (strict)"("Visible"=w282) -> ()  [unwired: 2 in, 2 out]
          }
          frame "Analog Out", "Motor", "PWM" {
            w288 = FALSE ("Visible")
            n153 = case shown="\"Analog Out\"" w287 {
              tunnel: [1.0 ("Value") -1.0 ("Value") 0.0 ("Value")] -> w286
              tunnel: [255.0 ("Value") 1.0 ("Value") 5.0 ("Value")] -> w285
              tunnel: [128.0 ("Value") 0.0 ("Value") 0.0 ("Value")] -> w284
              tunnel: [64.0 ("Value") 0.5 ("Value") 1.0 ("Value")] -> w283
              frame "PWM" {
              }
              frame "Motor", Default {
              }
              frame "Analog Out" {
              }
            }
            n154 = property on="Motor" class="Clust (strict)"("Visible"=TRUE) -> ()  [unwired: 2 in, 2 out]
            n155 = property on="Value" class="Slide (strict)"("Value"=w284, "Scale.Minimum"=w286, "Scale.Maximum"=w285, "Scale.Increment"=w283) -> ()  [unwired: 2 in, 2 out]
            n156 = property on="On/Off" class="Bool (strict)"("Visible"=w288) -> ()  [unwired: 2 in, 2 out]
            n157 = property on="Test Slider" class="Slide (strict)"("Visible"=w288) -> ()  [unwired: 2 in, 2 out]
            n158 = property on="Test Ring" class="Ring (strict)"("Visible"=w288) -> ()  [unwired: 2 in, 2 out]
            n159 = property on="Rev/Fwd" class="Clust (strict)"("Visible"=w288) -> ()  [unwired: 2 in, 2 out]
          }
          frame "Servo" {
            w304 = FALSE ("Visible")
            n160 = call <vilib>:"NT Read Number.vi"("Name"=w306) -> ("Numeric"=w305:dbl)  [unwired: 9 in, 1 out]
            n161 = property on="Test Slider" class="Slide (strict)"("Visible"=TRUE, "Scale.Maximum"=170.0 ("Scale.Range:Maximum")) -> ()  [unwired: 2 in, 2 out]
            n162 = local write "Test Slider"(w305) -> ()
            n163 = property on="Motor" class="Clust (strict)"("Visible"=w304) -> ()  [unwired: 2 in, 2 out]
            n164 = property on="Rev/Fwd" class="Clust (strict)"("Visible"=w304) -> ()  [unwired: 2 in, 2 out]
            n165 = property on="On/Off" class="Bool (strict)"("Visible"=w304) -> ()  [unwired: 2 in, 2 out]
            n166 = property on="Test Ring" class="Ring (strict)"("Visible"=w304) -> ()  [unwired: 2 in, 2 out]
          }
          frame "Relay", "Solenoid" {
            w307 = FALSE ("Visible")
            n167 = property on="Motor" class="Clust (strict)"("Visible"=w307) -> ()  [unwired: 2 in, 2 out]
            n168 = property on="Test Slider" class="Slide (strict)"("Visible"=w307) -> ()  [unwired: 2 in, 2 out]
            n169 = Search and Replace String(input string=w308, search string="/Value  **", replace string="/Direction") -> (result string=w314:string)  [unwired: 5 in, 3 out]
            n170 = property on="Test Ring" class="Ring (strict)"("Visible"=w307) -> ()  [unwired: 2 in, 2 out]
            n171 = call <vilib>:"NT Read String.vi"("Name"=w314) -> ("String"=w312:string)  [unwired: 9 in, 1 out]
            n172 = Equal?(x="Both directions", y=w312) -> (x = y?=w310:bool)
            n173 = Not(x=w310) -> (.not. x?=w311:bool)
            n174 = property on="Rev/Fwd" class="Clust (strict)"("Visible"=w310) -> ()  [unwired: 2 in, 2 out]
            n175 = property on="On/Off" class="Bool (strict)"("Visible"=w311, "Caption.Text"=w309) -> ()  [unwired: 2 in, 2 out]
          }
          frame "Compressor", "Digital Out" {
            w317 = FALSE ("Visible")
            # "Get direction and finish"
            n176 = property on="Motor" class="Clust (strict)"("Visible"=w317) -> ()  [unwired: 2 in, 2 out]
            n177 = property on="Test Slider" class="Slide (strict)"("Visible"=w317) -> ()  [unwired: 2 in, 2 out]
            n178 = property on="Test Ring" class="Ring (strict)"("Visible"=w317) -> ()  [unwired: 2 in, 2 out]
            n179 = property on="On/Off" class="Bool (strict)"("Visible"=TRUE, "Caption.Text"=w318) -> ()  [unwired: 2 in, 2 out]
            n180 = property on="Rev/Fwd" class="Clust (strict)"("Visible"=FALSE) -> ()  [unwired: 2 in, 2 out]
          }
          frame "Camera" {
            n181 = call <vilib>:"Get Last Path Segment.vi"("String in"=w325) -> ("String out"=w326:string)  [unwired: 10 in]
            n182 = property on="On/Off" class="Bool (strict)"("Visible"=FALSE) -> ()  [unwired: 2 in, 2 out]
            n183 = property on="Motor" class="Clust (strict)"("Visible"=FALSE) -> ()  [unwired: 2 in, 2 out]
            n184 = property on="Rev/Fwd" class="Clust (strict)"("Visible"=FALSE) -> ()  [unwired: 2 in, 2 out]
            n185 = case shown="\"White Balance  **\"" w326 {
              tunnel: w325 -> [w332 w341 w350 w359 w368 _ w374]
              tunnel: w324 -> [w330 w338 w347 w356 w365 _ _]
              frame "Size  **" {
                n186 = Index Array(array=w330) -> (element=w329:cluster{string[]})  [unwired: 1 in]
                n187 = call <vilib>:"NT Read String.vi"("Name"=w332) -> ("String"=w331:string)  [unwired: 9 in, 1 out]
                n188 = Unbundle(w329) -> (w327:string[])
                n189 = Match First String(2:w327, 3:w331) -> (0:w328:i32)  [unwired: 1 out]
                n190 = property on="Test Ring" class="Ring (strict)"("Value"=w328, "Strings []"=w327) -> ()  [unwired: 2 in, 2 out]
                n191 = property on="Test Ring" class="Ring (strict)"("Visible"=TRUE) -> ()  [unwired: 2 in, 2 out]
                n192 = property on="Test Slider" class="Slide (strict)"("Visible"=FALSE) -> ()  [unwired: 2 in, 2 out]
              }
              frame "White Balance  **" {
                n193 = Index Array(array=w338, index=1) -> (element=w339:cluster{string[]})
                n194 = call <vilib>:"NT Read String.vi"("Name"=w341) -> ("String"=w340:string)  [unwired: 9 in, 1 out]
                n195 = Unbundle(w339) -> (w336:string[])
                n196 = Match First String(2:w336, 3:w340) -> (0:w335:i32)  [unwired: 1 out]
                n197 = property on="Test Ring" class="Ring (strict)"("Value"=w335, "Strings []"=w336) -> ()  [unwired: 2 in, 2 out]
                n198 = property on="Test Ring" class="Ring (strict)"("Visible"=TRUE) -> ()  [unwired: 2 in, 2 out]
                n199 = property on="Test Slider" class="Slide (strict)"("Visible"=FALSE) -> ()  [unwired: 2 in, 2 out]
              }
              frame "Exposure  **" {
                n200 = Index Array(array=w347, index=2) -> (element=w348:cluster{string[]})
                n201 = call <vilib>:"NT Read String.vi"("Name"=w350) -> ("String"=w349:string)  [unwired: 9 in, 1 out]
                n202 = Unbundle(w348) -> (w344:string[])
                n203 = Match First String(2:w344, 3:w349) -> (0:w345:i32)  [unwired: 1 out]
                n204 = property on="Test Ring" class="Ring (strict)"("Value"=w345, "Strings []"=w344) -> ()  [unwired: 2 in, 2 out]
                n205 = property on="Test Ring" class="Ring (strict)"("Visible"=TRUE) -> ()  [unwired: 2 in, 2 out]
                n206 = property on="Test Slider" class="Slide (strict)"("Visible"=FALSE) -> ()  [unwired: 2 in, 2 out]
              }
              frame "Exposure Priority  **" {
                n207 = Index Array(array=w356, index=3) -> (element=w357:cluster{string[]})
                n208 = call <vilib>:"NT Read String.vi"("Name"=w359) -> ("String"=w358:string)  [unwired: 9 in, 1 out]
                n209 = Unbundle(w357) -> (w353:string[])
                n210 = Match First String(2:w353, 3:w358) -> (0:w354:i32)  [unwired: 1 out]
                n211 = property on="Test Ring" class="Ring (strict)"("Value"=w354, "Strings []"=w353) -> ()  [unwired: 2 in, 2 out]
                n212 = property on="Test Ring" class="Ring (strict)"("Visible"=TRUE) -> ()  [unwired: 2 in, 2 out]
                n213 = property on="Test Slider" class="Slide (strict)"("Visible"=FALSE) -> ()  [unwired: 2 in, 2 out]
              }
              frame "Color Enable  **" {
                n214 = Index Array(array=w365, index=4) -> (element=w366:cluster{string[]})
                n215 = call <vilib>:"NT Read String.vi"("Name"=w368) -> ("String"=w367:string)  [unwired: 9 in, 1 out]
                n216 = Unbundle(w366) -> (w362:string[])
                n217 = Match First String(2:w362, 3:w367) -> (0:w363:i32)  [unwired: 1 out]
                n218 = property on="Test Ring" class="Ring (strict)"("Value"=w363, "Strings []"=w362) -> ()  [unwired: 2 in, 2 out]
                n219 = property on="Test Ring" class="Ring (strict)"("Visible"=TRUE) -> ()  [unwired: 2 in, 2 out]
                n220 = property on="Test Slider" class="Slide (strict)"("Visible"=FALSE) -> ()  [unwired: 2 in, 2 out]
              }
              frame Default {
                n221 = property on="Test Ring" class="Ring (strict)"("Visible"=FALSE) -> ()  [unwired: 2 in, 2 out]
                n222 = property on="Test Slider" class="Slide (strict)"("Visible"=FALSE) -> ()  [unwired: 2 in, 2 out]
              }
              frame "Brightness  **", "Color Level  **", "Compression  **", "FPS  **", "Sharpness  **" {
                n223 = call <vilib>:"NT Read Number.vi"("Name"=w374) -> ("Numeric"=w373:dbl)  [unwired: 9 in, 1 out]
                n224 = local write "Test Slider"(w373) -> ()
                n225 = property on="Test Slider" class="Slide (strict)"("Visible"=TRUE, "Scale.Maximum"=100.0 ("Scale.Range:Maximum")) -> ()  [unwired: 2 in, 2 out]
                n226 = property on="Test Ring" class="Ring (strict)"("Visible"=FALSE) -> ()  [unwired: 2 in, 2 out]
              }
            }
          }
        }
        n227 = property on="Progress" class="Clust (strict)"("Visible"=FALSE) -> ()  [unwired: 2 in, 2 out]
      }
      event "Test Name": Mouse Enter {
        # "Populate the ring with the list of tests"
        n228 = event-data() -> ()  [unwired: 1 in, 1 out]
        n229 = call <vilib>:"NT Read String Array.vi"("Name"="TestMode/TestList") -> ("String Array"=w382:string[])  [unwired: 9 in, 1 out]
        n230 = Build Array (concatenate)("Select the test to run...", w382) -> (w381:string[])
        n231 = property on="Test Name" class="Ring (strict)"("Strings []"=w381) -> ()  [unwired: 2 in, 2 out]
      }
      event "Test Name": Value Change {
        w384 = FALSE ("Visible")
        # "Tell the robot the test name to run"
        n232 = event-data() -> ("NewVal"=w388:u16)  [unwired: 1 in]
        n233 = property on="Test Name" class="Ring (strict)"() -> ("Strings []"=w389:string[])  [unwired: 2 in, 2 out]
        n234 = local write "Progress"(T5 {"Test Progress"=0, "Test Progress Text"=""} ("Progress")) -> ()
        n235 = Index Array(array=w389, index=w388) -> (element=w387:string)
        n236 = call <vilib>:"NT Write String.vi"("String"=w387, "Name"="TestMode/TestName") -> ()  [unwired: 9 in, 1 out]
        n237 = property on="Progress" class="Clust (strict)"("Visible"=TRUE) -> ()  [unwired: 2 in, 2 out]
        n238 = property on="Motor" class="Clust (strict)"("Visible"=w384) -> ()  [unwired: 2 in, 2 out]
        n239 = property on="Test Slider" class="Slide (strict)"("Visible"=w384) -> ()  [unwired: 2 in, 2 out]
        n240 = property on="On/Off" class="Bool (strict)"("Visible"=w384) -> ()  [unwired: 2 in, 2 out]
        n241 = property on="Rev/Fwd" class="Clust (strict)"("Visible"=w384) -> ()  [unwired: 2 in, 2 out]
        n242 = property on="Test Ring" class="Ring (strict)"("Visible"=w384) -> ()  [unwired: 2 in, 2 out]
      }
      event "Select Auto": Mouse Enter {
        # "Populate the combo box with the list of autonomous options"
        n243 = event-data() -> ()  [unwired: 1 in, 1 out]
        n244 = call <vilib>:"NT Read String Array.vi"("Name"="Auto List") -> ("String Array"=w391:string[])  [unwired: 9 in, 1 out]
        n245 = property on="Select Auto" class="CmbBox"("Strings[]"=w391) -> ()  [unwired: 2 in, 2 out]
      }
      event "Select Auto": Value Change {
        # "User modified the Auto Selection. Write to NT variable so robot knows."
        n246 = event-data() -> ("NewVal"=w394:string)  [unwired: 1 in]
        n247 = call <vilib>:"NT Write String.vi"("String"=w394, "Name"="Auto Selector") -> ()  [unwired: 9 in, 1 out]
      }
      event "Command Selection": Value Change {
        # "Get the params and show in table"
        n248 = event-data() -> ("NewVal"=w400:i32)  [unwired: 1 in]
        n249 = property on="Command Selection" class="MCListbox (strict)"() -> ("ItemNames"=w398:string[][])  [unwired: 2 in, 2 out]
        n250 = call <vilib>:"WPI_DashboardUpdate Command Params.vi"("NewVal"=w400, "Commands"=w398, "Param Tbl"=w399) -> ()  [unwired: 8 in, 1 out]
      }
      event "Execute Command": Value Change {
        # "Started one, Unique ID holds\nresponse"
        n251 = event-data() -> ()  [unwired: 1 in, 1 out]
        n252 = property on="Command Selection" class="MCListbox (strict)"() -> ("ItemNames"=w411:string[][])  [unwired: 2 in, 2 out]
        n253 = Index Array(array=w411, index (row)="Command Selection", index (col)=0) -> (element=w409:string)
        n254 = call <vilib>:"Invoke Commands.vi"("Command Params"="Command Params", "Function Name"=w409) -> ("Params"=w405:u8, "Started"=w404:bool)  [unwired: 7 in, 1 out]
        n255 = Array Subset(array="Command Params", length (row)=w405) -> (w406:string[][])  [unwired: 3 in]
        n256 = Select(t="Executing" ("Cmd Status"), s=w404, f="" ("Cmd Status")) -> (s? t:f=→"Cmd Status":string)
      }
      event "Command Selection": Double Click {
        n257 = event-data() -> ("Row"=w419:i32)  [unwired: 1 in]
        n258 = property on="Command Selection" class="MCListbox (strict)"() -> ("ItemNames"=w422:string[][])  [unwired: 2 in, 2 out]
        n259 = local read "Command Params"() -> (w418:string[][])
        n260 = Index Array(array=w422, index (row)=w419, index (col)=0) -> (element=w420:string)
        n261 = call <vilib>:"Invoke Commands.vi"("Command Params"=w418, "Function Name"=w420) -> ("Params"=w417:u8, "Started"=w412:bool)  [unwired: 7 in, 1 out]
        n262 = Array Subset(array=w418, length (row)=w417) -> (w416:string[][])  [unwired: 3 in]
        n263 = Select(t="Executing" ("Cmd Status"), s=w412, f="" ("Cmd Status")) -> (s? t:f=w413:string)
        n264 = local write "Cmd Status"(w413) -> ()
      }
      event "CheckList": Double Click {
        # "Shift clears all"
        # "Update symbols on the listbox"
        n265 = event-data() -> ("PlatMods.Shift"=w424:bool, "Row"=w426:i32)  [unwired: 1 in]
        n266 = case shown="False" w424 {
          tunnel: w426 -> [w430 _]
          tunnel: 1 -> [w429 _]
          frame False {
            n267 = property on="CheckList" class="LstBox (strict)"() -> ("Item Symbols"=w428:i32[])  [unwired: 2 in, 2 out]
            n268 = Replace Array Subset(array=w428, new element=w429, index=w430) -> (w427:i32[])
            n269 = property on="CheckList" class="LstBox (strict)"("Item Symbols"=w427) -> ()  [unwired: 2 in, 2 out]
          }
          frame True {
            w431 = 0 ("Top Row")
            n270 = property on="CheckList" class="LstBox (strict)"() -> ("Number of Rows"=w433:u32)  [unwired: 2 in, 2 out]
            n271 = Initialize Array(0, w433) -> (w432:i32[])
            n272 = property on="CheckList" class="LstBox (strict)"("Top Row"=w431, "Value"=w431, "Item Symbols"=w432) -> ()  [unwired: 2 in, 2 out]
          }
        }
      }
      event "CheckList": Key Down {
        # "Update symbols on the listbox\nLeft and right keys check and uncheck"
        n273 = event-data() -> ("VKey"=w437:T20)  [unwired: 1 in]
        n274 = case shown="\"Left\", \"Right\"" w437 {
          selector: w437 -> [w442 _]
          tunnel: eventvkey."Left" ("VKey") -> [w440 _]
          frame "Left", "Right" {
            n275 = Equal?(x=w440, y=w442) -> (x = y?=w441:bool)
            n276 = Select(t=0, s=w441, f=1) -> (s? t:f=w443:i32)
            n277 = property on="CheckList" class="LstBox (strict)"() -> ("Item Symbols"=w446:i32[])  [unwired: 2 in, 2 out]
            n278 = Replace Array Subset(array=w446, new element=w443, index="CheckList") -> (w445:i32[])
            n279 = property on="CheckList" class="LstBox (strict)"("Item Symbols"=w445) -> ()  [unwired: 2 in, 2 out]
          }
          frame Default {
          }
        }
      }
      event "Motor.Enable": Value Change {
        # "When the test mode otor enable helper is set, update that\ntree row item's value"
        n280 = event-data() -> ("NewVal"=w452:bool)  [unwired: 1 in]
        n281 = Unbundle("Motor") -> ("Value"=w451:dbl)  [unwired: 1 out]
        n282 = Select(t=w451, s=w452, f=0.0) -> (s? t:f=w449:dbl)
        n283 = call <vilib>:"NT Write Number.vi"("Numeric"=w449, "Name"=w448) -> ()  [unwired: 9 in, 1 out]
      }
      event "Test Slider": Value Change {
        # "When the test mode slider helper is set, update that\ntree row item's value"
        n284 = event-data() -> ("NewVal"=w455:dbl)  [unwired: 1 in]
        n285 = call <vilib>:"NT Write Number.vi"("Numeric"=w455, "Name"=w456) -> ()  [unwired: 9 in, 1 out]
      }
      event "On/Off": Value Change {
        # "When the test mode on/off helper value is set, update that\ntree row item's value"
        n286 = event-data() -> ("NewVal"=w460:bool)  [unwired: 1 in]
        n287 = Boolean To (0,1)(Boolean=w460) -> (0, 1=w459:i16)
        n288 = call <vilib>:"NT Write Number.vi"("Numeric"=w459, "Name"=w458) -> ()  [unwired: 9 in, 1 out]
      }
      event "Rev/Fwd": Value Change {
        # "When the test mode helper value for relays is set, update that\ntree row item's value"
        n289 = event-data() -> ("NewVal.Forward"=w468:bool, "NewVal.Reverse"=w467:bool)  [unwired: 1 in]
        n290 = Boolean To (0,1)(Boolean=w468) -> (0, 1=w464:i16)
        n291 = Boolean To (0,1)(Boolean=w467) -> (0, 1=w466:i16)
        n292 = Negate(x=w466) -> (-x=w465:i16)
        n293 = Add(x=w464, y=w465) -> (x+y=w463:i16)
        n294 = call <vilib>:"NT Write Number.vi"("Numeric"=w463, "Name"=w462) -> ()  [unwired: 9 in, 1 out]
      }
      event "Test Ring": Value Change {
        # "When a test mode helper value is selected from the ring,\nset the tree item's variable to the string value"
        n295 = event-data() -> ("NewVal"=w472:u16)  [unwired: 1 in]
        n296 = property on="Test Ring" class="Ring (strict)"() -> ("Strings []"=w473:string[])  [unwired: 2 in, 2 out]
        n297 = Index Array(array=w473, index=w472) -> (element=w471:string)
        n298 = call <vilib>:"NT Write String.vi"("String"=w471, "Name"=w470) -> ()  [unwired: 9 in, 1 out]
      }
      event "Rec Mode": Value Change {
        # "Update globals for recording mode and path to read log from.\nClear when logging and let NetworkTables set path for vision to\nuse."
        n299 = event-data() -> ("NewVal"=w482:enum32{"Stop", "Record", "Playback"})  [unwired: 1 in]
        n300 = global write "WPI_DashboardLogging Global.vi" "Logging Filename"(path "") -> ()
        n301 = global write "WPI_DashboardLogging Global.vi" "Recording"(w482) -> ()
        n302 = case shown="\"Playback\"" w482 {
          tunnel: w481 -> [_ w484 w491]
          tunnel: [_ _ w490] -> w479
          tunnel: [_ _ w489] -> _
          tunnel: w477 -> [_ _ w487]
          tunnel: cluster{i32, i32} {-250, 170} -> [_ _ w486]
          tunnel: w475 -> [_ _ w485]
          frame Default {
          }
          frame "Stop", "Record" {
            # "Place Window too"
            n303 = invoke class="VI" method="FP.Close"(reference=w484) -> (reference out=w483:refnum<vi>)  [unwired: 2 in, 2 out]
            n304 = invoke class="VI" method="Abort VI"(reference=w483) -> ()  [unwired: 2 in, 3 out]
          }
          frame "Playback" {
            n305 = call "Open Playback Panel.vi"("Offset"=w486, "DB VI Ref"=w487, "Playback in"=w491) -> ("Playback out"=w488:refnum<vi>)  [unwired: 8 in]
            n306 = register-events(w488, w485) -> (reference out=w490:refnum<event-registration>, error out=w489:errorcluster)  [unwired: 2 in]
          }
        }
        n307 = call <vilib>:"WPI_DashboardNT Log FieldName Cache.vi"("Operation"=enum16{"Lookup/Add", "Index", "Clear"}."Clear") -> ()  [unwired: 8 in, 3 out]
      }
      event Panel Close {
        w493 = enum32{"Stop", "Record", "Playback"}."Stop" ("Rec Mode")
        # "Playback window has been closed, abort"
        n308 = event-data() -> ()  [unwired: 1 in, 4 out]
        n309 = local write "Rec Mode"(w493) -> ()
        n310 = global write "WPI_DashboardLogging Global.vi" "Recording"(w493) -> ()
      }
      event Panel Close {
        # "Abort playback window and ourself"
        n311 = event-data() -> ()  [unwired: 1 in, 4 out]
        n312 = invoke class="VI" method="FP.Close"(reference=w497) -> (reference out=w496:refnum<vi>)  [unwired: 2 in, 2 out]
        n313 = invoke class="VI" method="Abort VI"(reference=w496) -> (error out=w495:errorcluster)  [unwired: 2 in, 2 out]
        n314 = invoke class="VI" method="Abort VI"(error in=w495) -> ()  [unwired: 2 in, 3 out]
      }
      event User Event {
        n315 = event-data() -> ("IDs"=w504:cluster{"RPC field ID":u16, "Unique ID":u16}, "String"=w503:string)  [unwired: 1 in]
        n316 = Bundle("IDs"=w504, "String"=w503) -> (w502:T10)  [unwired: 1 in]
        n317 = call <vilib>:"Retrieve RPC Response.vi"("RPC Response"=w502) -> ("Output"=w500:string[][])  [unwired: 10 in]
        n318 = Build Array (concatenate)(w498, w500) -> (w499:string[][])
        n319 = local write "Command Params"(w499) -> ()
        n320 = local write "Cmd Status"("" ("Cmd Status")) -> ()
      }
      event "Tree": Double Click {
        n321 = event-data() -> ("PlatMods"=w510:T23, "Tag"=w507:string)  [unwired: 1 in]
        n322 = Unbundle(w510) -> ("Shift"=w509:bool)  [unwired: 4 out]
        n323 = String Subset(string=w507, length (rest)=1 ("length (rest)")) -> (substring=w506:string)  [unwired: 1 in]
        n324 = Not(x=w509) -> (.not. x?=w508:bool)
        n325 = case shown="\"/\"" w506 {
          tunnel: w507 -> [_ w513]
          tunnel: w508 -> [_ w512]
          frame Default {
          }
          frame "/" {
            n326 = call <vilib>:"NT Update Persistence.vi"("Persistence"=w512, "Name"=w513) -> ()  [unwired: 9 in, 1 out]
          }
        }
      }
    }
  }
  n327 = while {
    tunnel: w61 -> [w515]
    i -> [w518]
    stop <- FALSE stop-if-true
    n328 = Wait (ms)(milliseconds to wait=u32 100) -> ()  [unwired: 1 out]
    n329 = case shown="\"Playback\"" "Rec Mode" {
      tunnel: w518 -> [_ _ w533]
      tunnel: [u32 2829099 ("Base Color") u32 11141120 ("Target Color") w522] -> w514
      frame "Stop", Default {
        # "Reset the color, extra updates don't cost much"
      }
      frame "Record" {
      }
      frame "Playback" {
        # "Playback"
        n330 = Quotient & Remainder(x=w533, y=u32 50 ("milliseconds to wait")) -> (x-y*floor(x/y)=w529:u32)  [unwired: 1 out]
        n331 = Divide(x=w529, y=u32 50 ("milliseconds to wait")) -> (x/y=w526:dbl)
        n332 = Multiply(x=6.283185307179586, y=w526) -> (x*y=w531:dbl)
        n333 = Sine(x=w531) -> (sin(x)=w530:dbl)
        n334 = Absolute Value(x=w530) -> (abs(x)=w523:dbl)
        n335 = call "Interpolate RGB Color.vi"("Proportion"=w523, "Target Color"=u32 30976, "Base Color"=u32 2829099) -> ("Result Color"=w522:u32)  [unwired: 8 in]
      }
    }
    n336 = property class="Pane"(reference=w515, "PaneColor"=w514) -> ()  [unwired: 1 in, 2 out]
  }
  n337 = property on="On/Off" class="Bool (strict)"("Visible"=w34) -> ()  [unwired: 2 in, 2 out]
  n338 = property on="Motor" class="Clust (strict)"("Visible"=w34) -> ()  [unwired: 2 in, 2 out]
  n339 = property on="Progress" class="Clust (strict)"("Visible"=w34) -> ()  [unwired: 2 in, 2 out]
  n340 = property on="Test Ring" class="Ring (strict)"("Visible"=w34) -> ()  [unwired: 2 in, 2 out]
  n341 = property on="Rev/Fwd" class="Clust (strict)"("Visible"=w34) -> ()  [unwired: 2 in, 2 out]
  n342 = while {
    tunnel: u16 1741 ("timeout ms (25000)") -> [w535]
    stop <- FALSE stop-if-true
    n343 = TCP Create Listener(10:w535) -> (0:w534:errorcluster, 3:w536:refnum<k5>)  [unwired: 4 in, 1 out]
    n344 = case shown="No Error" w534 {
      selector: w534 -> [w538 _]
      tunnel: w536 -> [w539 _]
      frame No Error {
        n345 = while {
          tunnel: w539 -> [w542]
          tunnel: w538 -> [w541]
          stop <- FALSE stop-if-true
          n346 = TCP Wait On Listener(8:w541, 11:w542) -> (0:w543:errorcluster, 4:w544:refnum<k5>)  [unwired: 2 in, 3 out]
          n347 = local write "TCP"(w544) -> ()
          n348 = case shown="No Error" w543 {
            frame No Error {
            }
            frame Error {
              n349 = Wait (ms)(milliseconds to wait=u32 1000) -> ()  [unwired: 1 out]
            }
          }
        }
      }
      frame Error {
        n350 = Wait (ms)(milliseconds to wait=u32 1000) -> ()  [unwired: 1 out]
      }
    }
  }
  n351 = local write "Command Selection"(u16 0 ("milliseconds to wait")) -> ()
  n352 = local write "Command Params"(string[][] [] ("Command Params")) -> ()
  n353 = global write "WPI_DashboardLogging Global.vi" "Recording"(w55) -> ()
  n354 = local write "Rec Mode"(w55) -> ()
  n355 = call <vilib>:"NT Write String.vi"("String"="Select Auto", "Name"="Auto Selector") -> ()  [unwired: 9 in, 1 out]
